vi "ETOI to ED.vi"(11 "Excluded Tests on Items":T1(array[cluster])) -> (3 "Exclusion Data":T2[](array[typedef]))   [LabVIEW 2020]
uses:
  <vilib>/addons/analyzer/_analyzerctrls.llb/VIAnCtl Exclusion Data.ctl
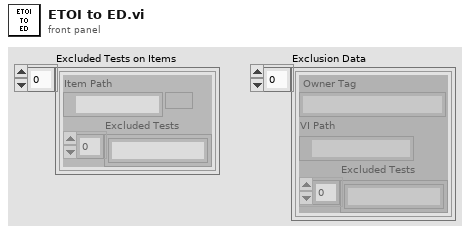
[diagram p1: front panel]
types:
  T1 = cluster{"Item Path":path, "Excluded Tests":string[]}[]
  T2 = typedef "VIAnCtl Exclusion Data.ctl" = cluster{"Owner Tag":string, "VI Path":path, "Excluded Tests":string[]}
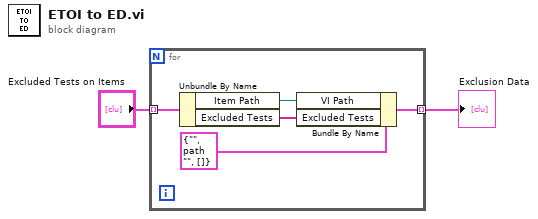
[diagram p0: block diagram]
diagram:
  n1 = for {
    tunnel: "Excluded Tests on Items" -> [w7] mode=indexing
    tunnel: [w3] -> w2 mode=indexing
    n2 = Unbundle By Name(w7) -> ("Item Path"=w5:path, "Excluded Tests"=w4:string[])
    n3 = Bundle By Name(cluster=T2 {"Owner Tag"="", "VI Path"=path "", "Excluded Tests"=[]} ("Data"), "VI Path"=w5, "Excluded Tests"=w4) -> (w3:T2)
  }
  "Exclusion Data" <- w2
